vi "Dashboard and Primary Interface.vi"() -> ()   [LabVIEW 2020]
uses:
  C:/Users/fg/Documents/UniversalRobots.vi/LabVIEW_2024/UnderAutomation.UniversalRobots/lib/UnderAutomation.UniversalRobots.dll
  LabVIEW_2024/UnderAutomation.UniversalRobots/lib/UnderAutomation.UniversalRobots.dll
panel:
  in  "disconnect SFTP":bool caption="Disconnect Sftp"
  out "Connected":bool
  out "EnumeratePrograms":string[](array[string])
  in  "Enumerate":bool
  in  "password":string
  in  "username":string
  in  "Connect SFTP":bool caption="Connect Sftp"
  in  "Program name":string
  in  "Start program":bool
  out "Powered on":bool
  in  "Script to execute":string
  in  "Send script":bool
  out "Z":dbl
  out "Y":dbl
  out "X":dbl
  in  "Robot IP":string
  out "Connect error":errorcluster
  in  "Power off":bool
  in  "Power on\nRelease brake":bool
  out "Connected":bool
  in  "Connect":bool
  # "1. Connect to the robot"
  # "2. Dashboard"
  # "3. Primary Interface"
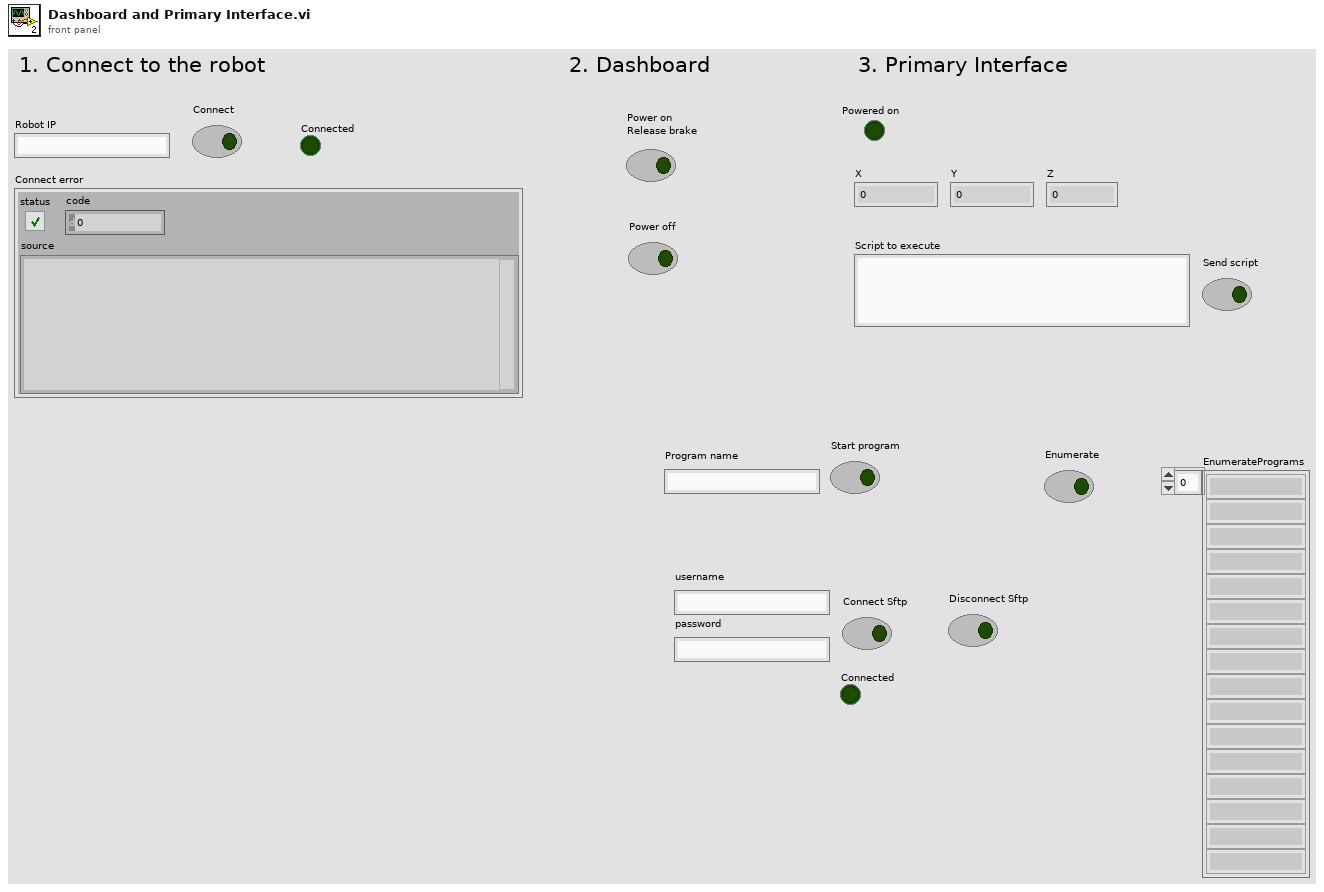
[diagram p1: front panel]
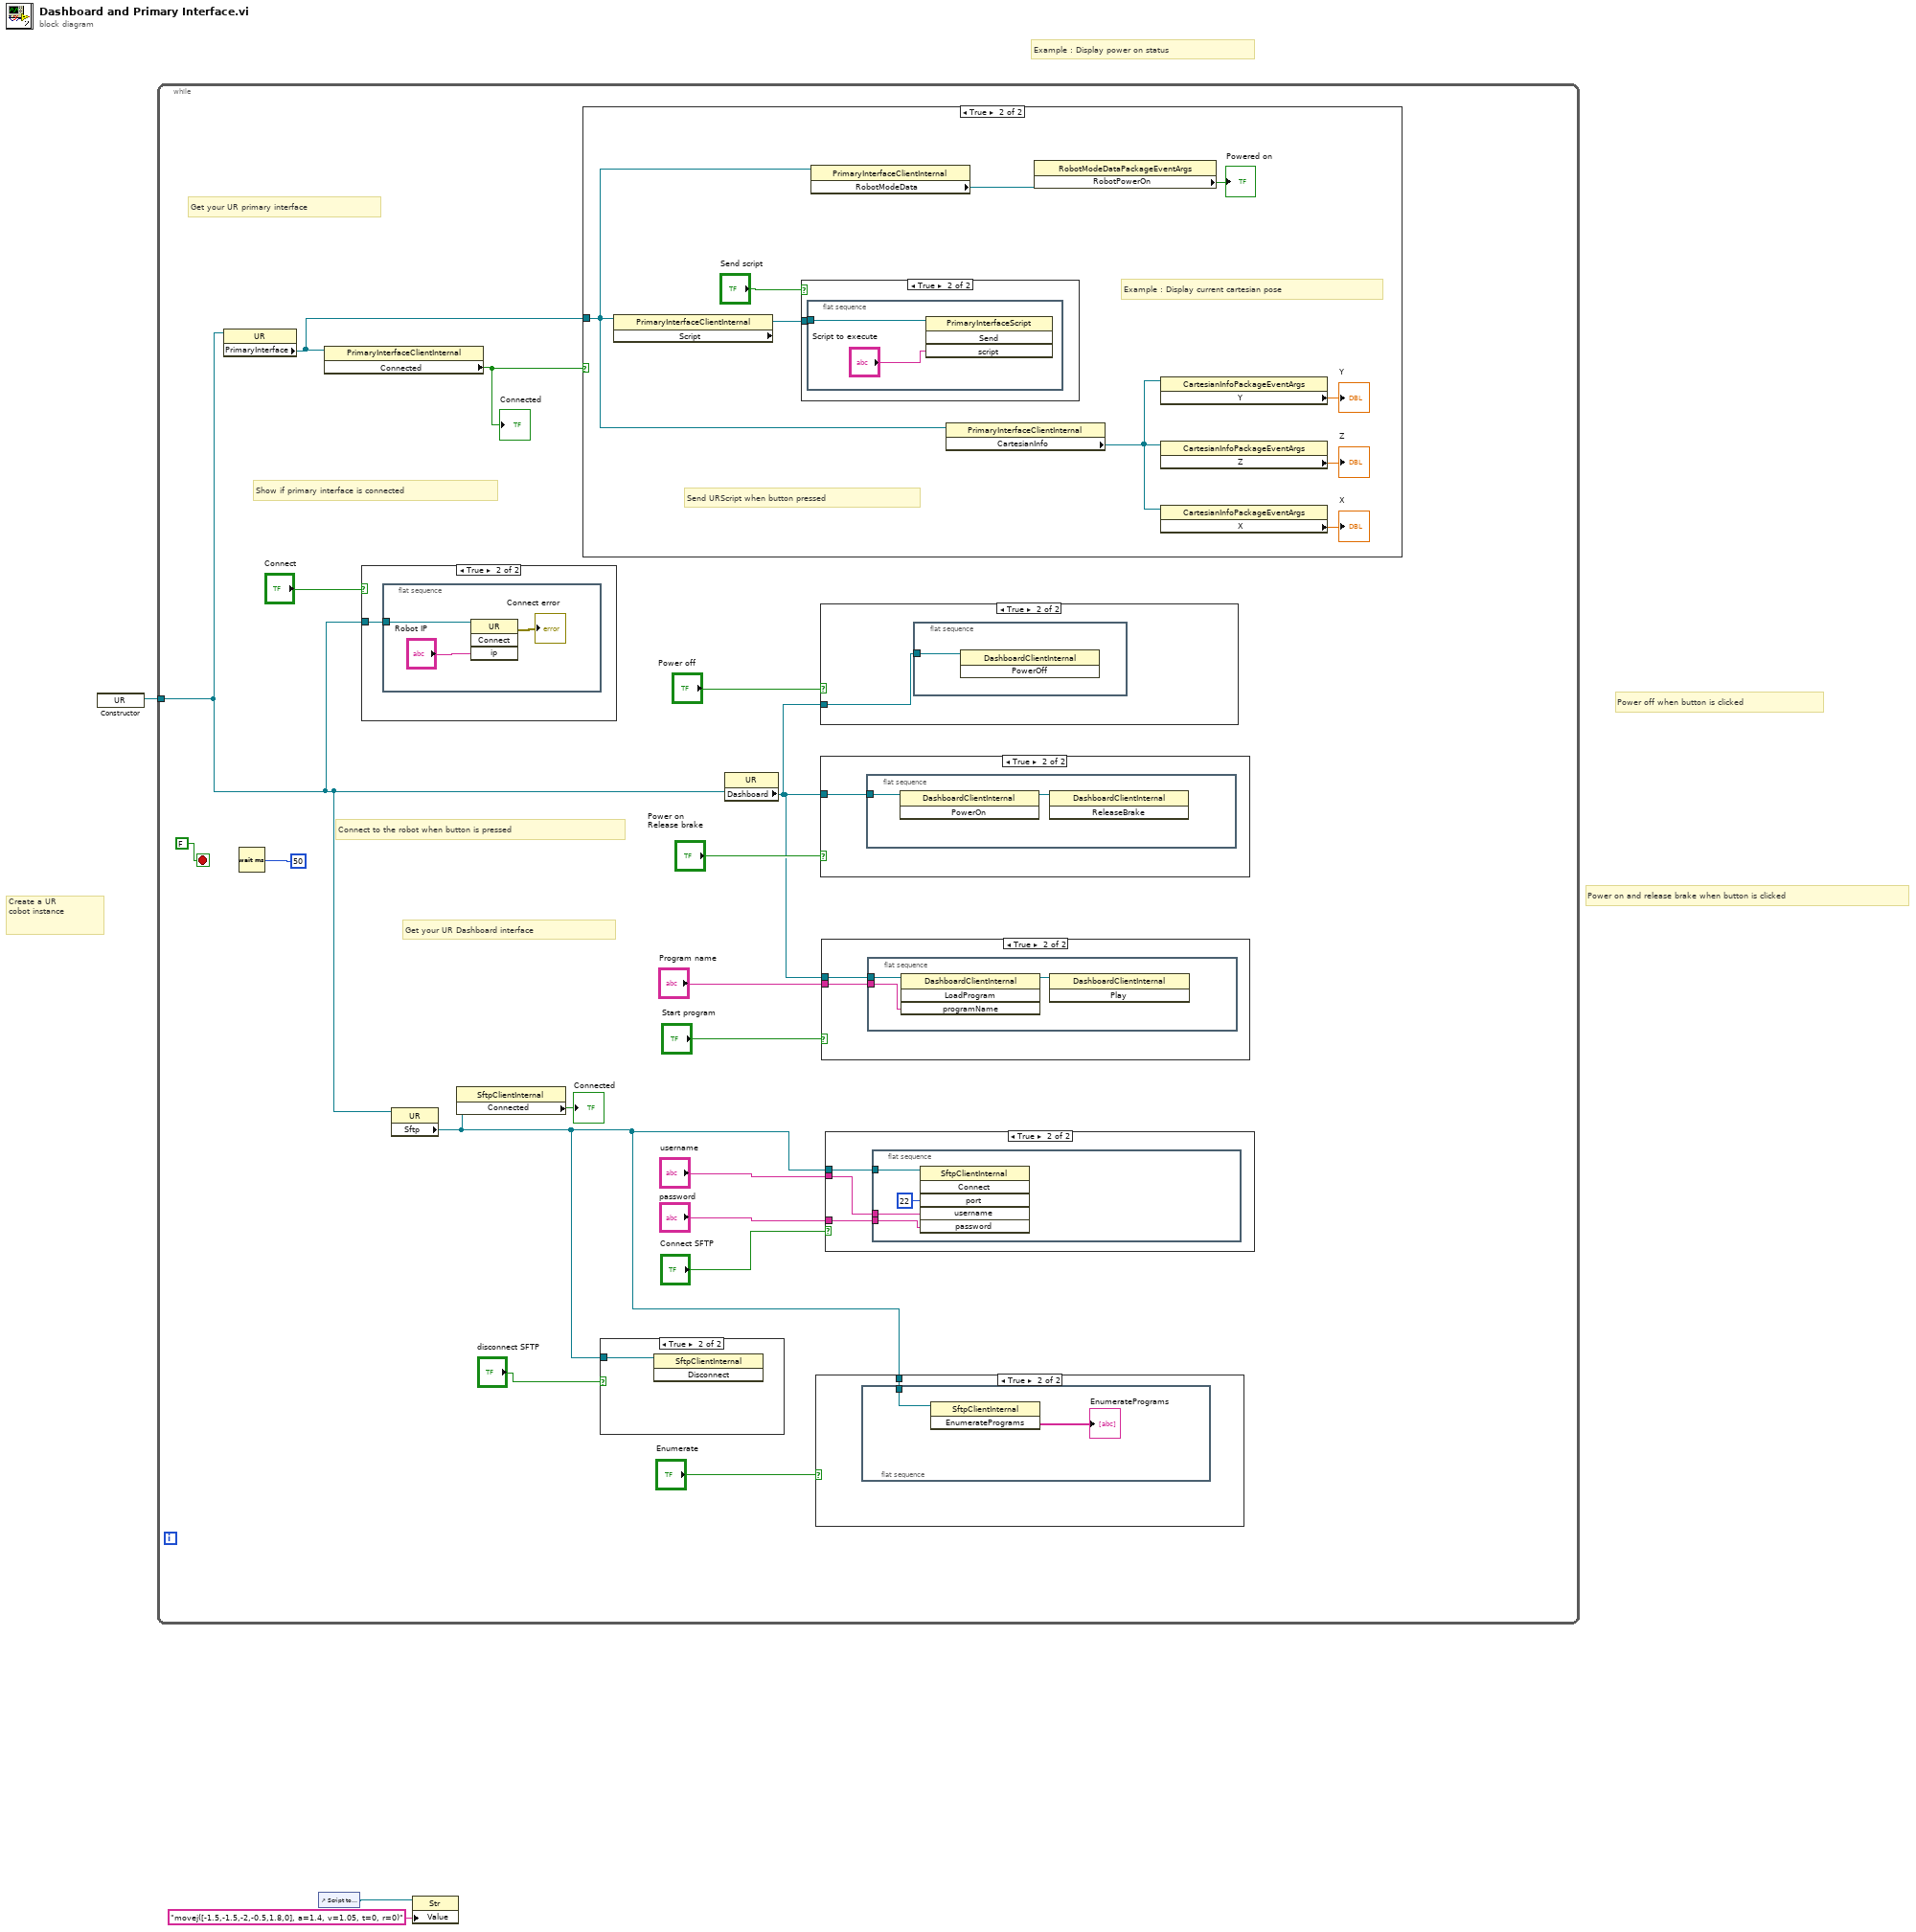
[diagram p0: block diagram]
diagram:
  # "Example : Display power on status"
  # "Create a UR\ncobot instance"
  # "Power off when button is clicked"
  # "Power on and release brake when button is clicked"
  n1 = constructor class="UR"() -> (reference out=w3:refnum<k24>)  [unwired: 3 in, 2 out]
  n2 = while {
    tunnel: w3 -> [w11]
    stop <- FALSE stop-if-true
    # "Get your UR Dashboard interface"
    # "Connect to the robot when button is pressed"
    # "Show if primary interface is connected"
    # "Get your UR primary interface"
    n3 = property class="UR"(reference=w11) -> ("PrimaryInterface"=w17:refnum<k24>)  [unwired: 1 in, 2 out]
    n4 = Wait (ms)(milliseconds to wait=u32 50) -> ()  [unwired: 1 out]
    n5 = property class="PrimaryInterfaceClientInternal"(reference=w17) -> ("Connected"=w16:bool)  [unwired: 1 in, 2 out]
    "Connected" <- w16
    n6 = case shown="True" "Connect" {
      tunnel: w11 -> [_ w55]
      frame False {
      }
      frame True {
        n7 = flat-sequence {
          tunnel: w55 -> [w57]
          frame #0 {
            n8 = invoke class="UR" method="Connect"(reference=w57, "ip"="Robot IP") -> (error out=→"Connect error":errorcluster)  [unwired: 2 in, 3 out]
          }
        }
      }
    }
    n9 = property class="UR"(reference=w11) -> ("Sftp"=w4:refnum<k24>)  [unwired: 1 in, 2 out]
    n10 = property class="SftpClientInternal"(reference=w4) -> ("Connected"=→"Connected":bool)  [unwired: 1 in, 2 out]
    n11 = case shown="True" w16 {
      tunnel: w17 -> [_ w38]
      frame False {
      }
      frame True {
        # "Send URScript when button pressed"
        # "Example : Display current cartesian pose"
        n12 = property class="PrimaryInterfaceClientInternal"(reference=w38) -> ("Script"=w45:refnum<k24>)  [unwired: 1 in, 2 out]
        n13 = case shown="True" "Send script" {
          tunnel: w45 -> [_ w47]
          frame False {
          }
          frame True {
            n14 = flat-sequence {
              tunnel: w47 -> [w49]
              frame #0 {
                n15 = invoke class="PrimaryInterfaceScript" method="Send"(reference=w49, "script"="Script to execute") -> ()  [unwired: 2 in, 4 out]
              }
            }
          }
        }
        n16 = property class="PrimaryInterfaceClientInternal"(reference=w38) -> ("RobotModeData"=w44:refnum<k24>)  [unwired: 1 in, 2 out]
        n17 = property class="PrimaryInterfaceClientInternal"(reference=w38) -> ("CartesianInfo"=w39:refnum<k24>)  [unwired: 1 in, 2 out]
        n18 = property class="RobotModeDataPackageEventArgs"(reference=w44) -> ("RobotPowerOn"=→"Powered on":bool)  [unwired: 1 in, 2 out]
        n19 = property class="CartesianInfoPackageEventArgs"(reference=w39) -> ("Y"=→"Y":dbl)  [unwired: 1 in, 2 out]
        n20 = property class="CartesianInfoPackageEventArgs"(reference=w39) -> ("Z"=→"Z":dbl)  [unwired: 1 in, 2 out]
        n21 = property class="CartesianInfoPackageEventArgs"(reference=w39) -> ("X"=→"X":dbl)  [unwired: 1 in, 2 out]
      }
    }
    n22 = case shown="True" "disconnect SFTP" {
      tunnel: w4 -> [_ w22]
      frame False {
      }
      frame True {
        n23 = invoke class="SftpClientInternal" method="Disconnect"(reference=w22) -> ()  [unwired: 2 in, 3 out]
      }
    }
    n24 = property class="UR"(reference=w11) -> ("Dashboard"=w13:refnum<k24>)  [unwired: 1 in, 2 out]
    n25 = case shown="True" "Enumerate" {
      tunnel: w4 -> [_ w23]
      frame False {
      }
      frame True {
        n26 = flat-sequence {
          tunnel: w23 -> [w25]
          frame #0 {
            n27 = invoke class="SftpClientInternal" method="EnumeratePrograms"(reference=w25) -> ("EnumeratePrograms"=→"EnumeratePrograms":string[])  [unwired: 2 in, 2 out]
          }
        }
      }
    }
    n28 = case shown="True" "Power off" {
      tunnel: w13 -> [_ w50]
      frame False {
      }
      frame True {
        n29 = flat-sequence {
          tunnel: w50 -> [w51]
          frame #0 {
            n30 = invoke class="DashboardClientInternal" method="PowerOff"(reference=w51) -> ()  [unwired: 2 in, 3 out]
          }
        }
      }
    }
    n31 = case shown="True" "Power on\nRelease brake" {
      tunnel: w13 -> [_ w52]
      frame False {
      }
      frame True {
        n32 = flat-sequence {
          tunnel: w52 -> [w54]
          frame #0 {
            n33 = invoke class="DashboardClientInternal" method="PowerOn"(reference=w54) -> (reference out=w53:refnum<k24>)  [unwired: 2 in, 2 out]
            n34 = invoke class="DashboardClientInternal" method="ReleaseBrake"(reference=w53) -> ()  [unwired: 2 in, 3 out]
          }
        }
      }
    }
    n35 = case shown="True" "Start program" {
      tunnel: w13 -> [_ w34]
      tunnel: "Program name" -> [_ w33]
      frame False {
      }
      frame True {
        n36 = flat-sequence {
          tunnel: w34 -> [w37]
          tunnel: w33 -> [w35]
          frame #0 {
            n37 = invoke class="DashboardClientInternal" method="LoadProgram"(reference=w37, "programName"=w35) -> (reference out=w36:refnum<k24>)  [unwired: 2 in, 3 out]
            n38 = invoke class="DashboardClientInternal" method="Play"(reference=w36) -> ()  [unwired: 2 in, 3 out]
          }
        }
      }
    }
    n39 = case shown="True" "Connect SFTP" {
      tunnel: w4 -> [_ w28]
      tunnel: "username" -> [_ w27]
      tunnel: "password" -> [_ w26]
      frame False {
      }
      frame True {
        n40 = flat-sequence {
          tunnel: w28 -> [w32]
          tunnel: w27 -> [w30]
          tunnel: w26 -> [w31]
          frame #0 {
            n41 = invoke class="SftpClientInternal" method="Connect"(reference=w32, "port"=22, "username"=w30, "password"=w31) -> ()  [unwired: 2 in, 6 out]
          }
        }
      }
    }
  }
  n42 = control-ref of="Script to execute"() -> (w2:refnum<vi>)
  n43 = property class="Str"(reference=w2, "Value"="movej([-1.5,-1.5,-2,-0.5,1.8,0], a=1.4, v=1.05, t=0, r=0)") -> ()  [unwired: 1 in, 2 out]
